vi "Decode IA_State.vi"(8 "error in (no error)":errorcluster, 11 "array":u8[](array[numeric])) -> (0 "error out":errorcluster, 3 "output cluster":T2)   [LabVIEW 2017]
uses:
  Util/Events/Events.ctl
panel:
  in  "?":T2={"Our_Robots"=[], "Events"={"Touch"=FALSE, "Ball out"=FALSE, "id touch"=0.0, "Ball out of \nVision"=FALSE, "Ball inside \nGoalie area"=FALSE, "Robot not responding"=FALSE, "Robots responding status"=[1.0, 1.0, 1.0, 1.0, 1.0, 1.0], "Enemy Ball \nPossession"=FALSE, "Pass State"=FALSE, "id end of pass"=0.0, "Kick"=FALSE, "Id ini Possession"=0.0, "Ball Possesion"=FALSE, "Id Possesion"=0.0}}
  out "array w/ subset deleted":u8[](array[numeric])
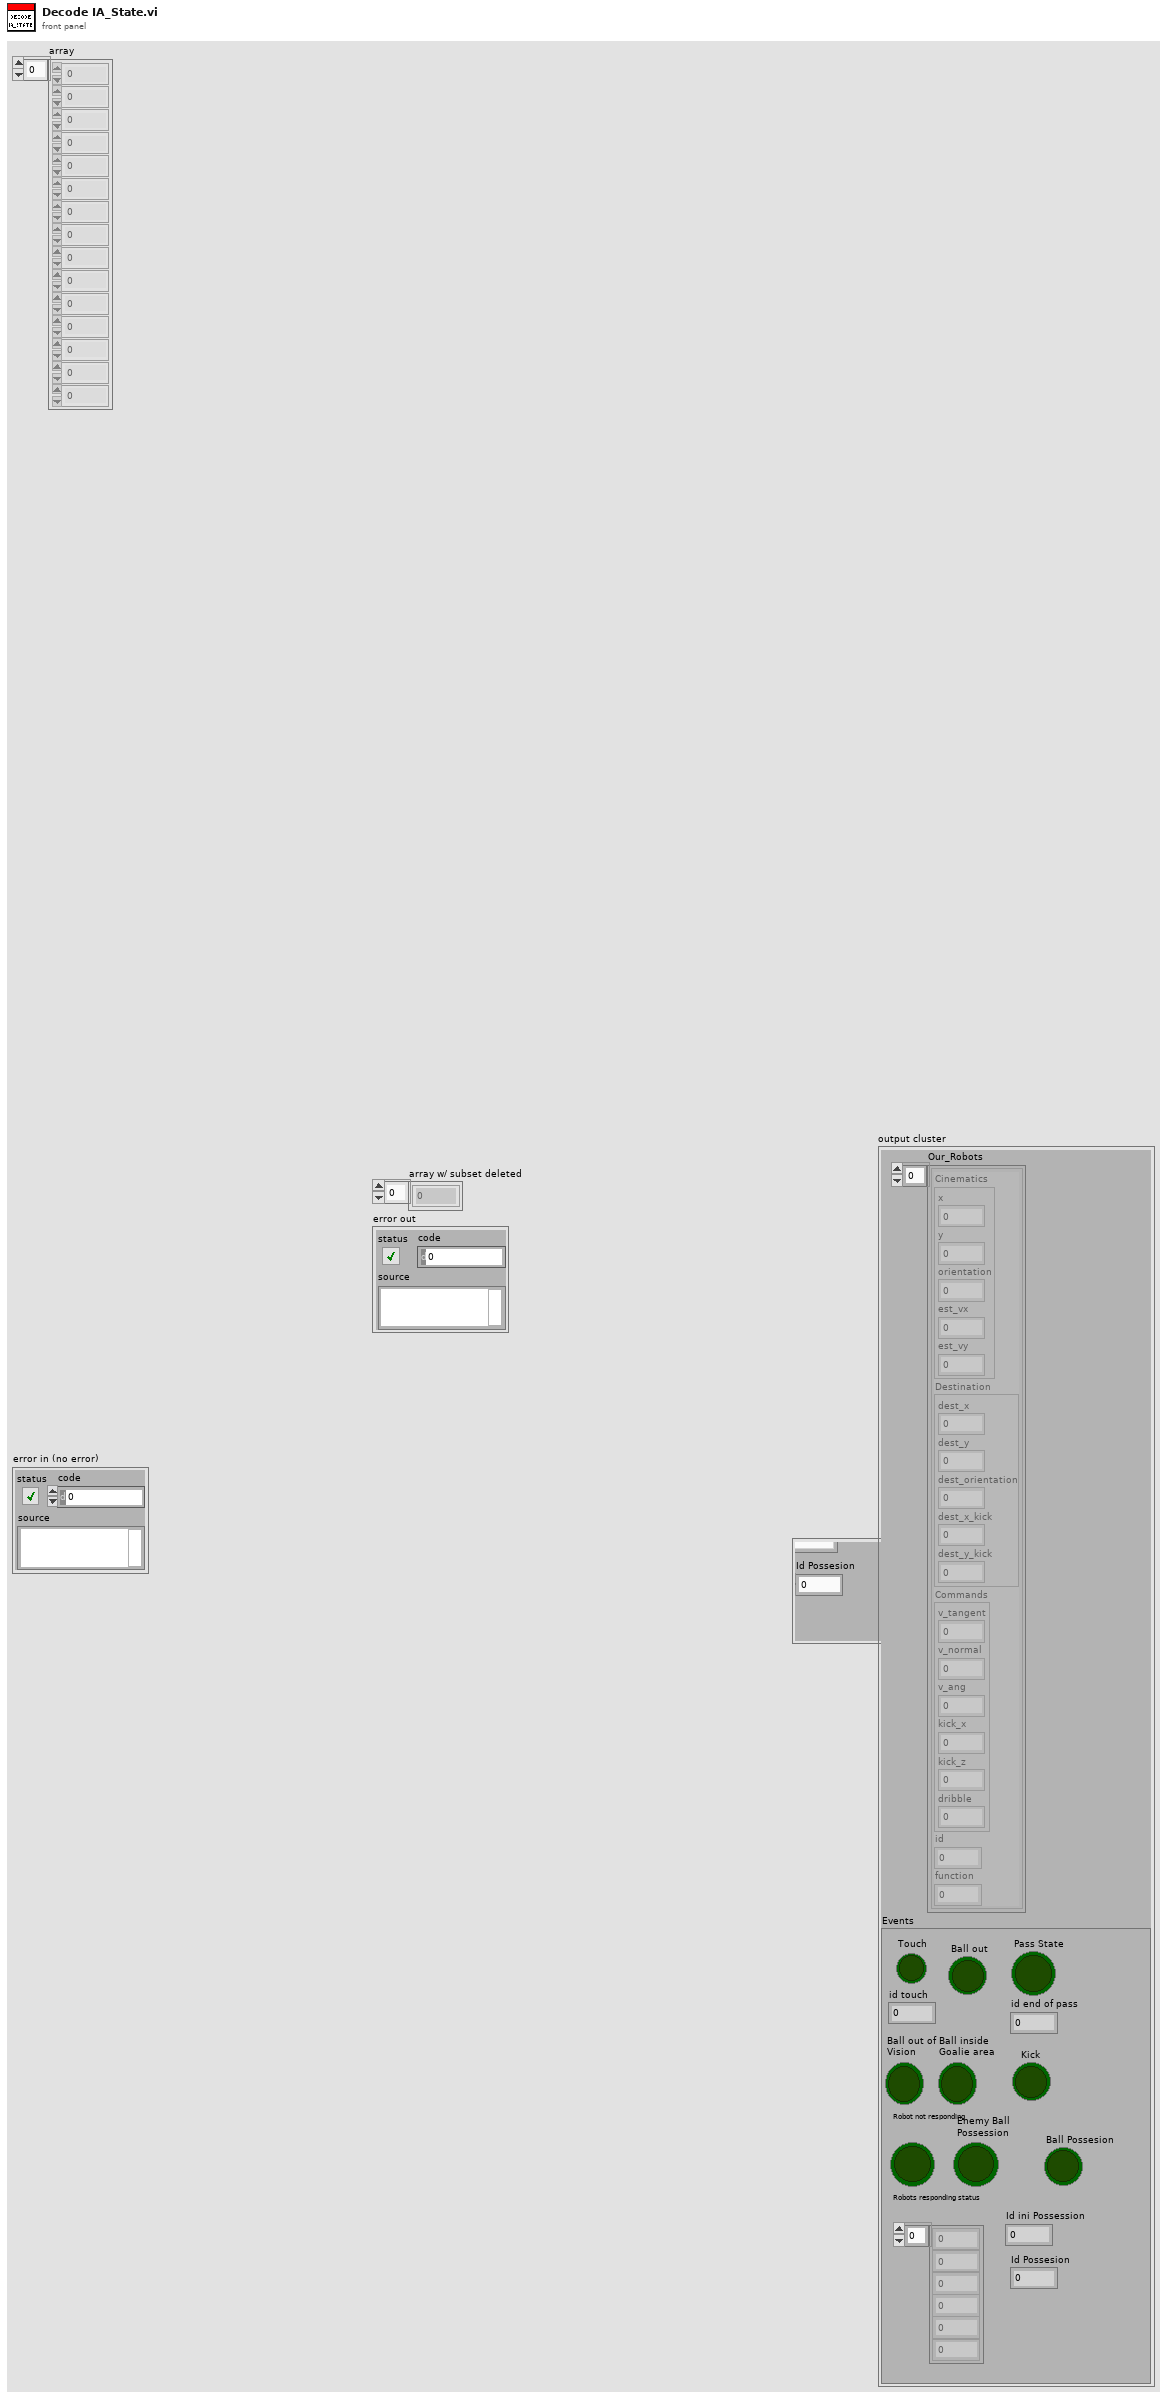
[diagram p1: front panel]
types:
  T1 = typedef "Events.ctl" = cluster{"Touch":bool, "Ball out":bool, "id touch":dbl, "Ball out of \nVision":bool, "Ball inside \nGoalie area":bool, "Robot not responding":bool, "Robots responding status":dbl[], "Enemy Ball \nPossession":bool, "Pass State":bool, "id end of pass":dbl, "Kick":bool, "Id ini Possession":dbl, "Ball Possesion":bool, "Id Possesion":dbl}
  T2 = cluster{"Our_Robots":cluster{"Cinematics":cluster{"x":dbl, "y":dbl, "orientation":dbl, "est_vx":dbl, "est_vy":dbl}, "Destination":cluster{"dest_x":dbl, "dest_y":dbl, "dest_orientation":dbl, "dest_x_kick":dbl, "dest_y_kick":dbl}, "Commands":cluster{"v_tangent":dbl, "v_normal":dbl, "v_ang":dbl, "kick_x":dbl, "kick_z":dbl, "dribble":u32}, "id":u32, "function":u32}[], "Events":T1}
  T3 = cluster{"Cinematics":cluster{"x":dbl, "y":dbl, "orientation":dbl, "est_vx":dbl, "est_vy":dbl}, "Destination":cluster{"dest_x":dbl, "dest_y":dbl, "dest_orientation":dbl, "dest_x_kick":dbl, "dest_y_kick":dbl}, "Commands":cluster{"v_tangent":dbl, "v_normal":dbl, "v_ang":dbl, "kick_x":dbl, "kick_z":dbl, "dribble":u32}, "id":u32, "function":u32}[]
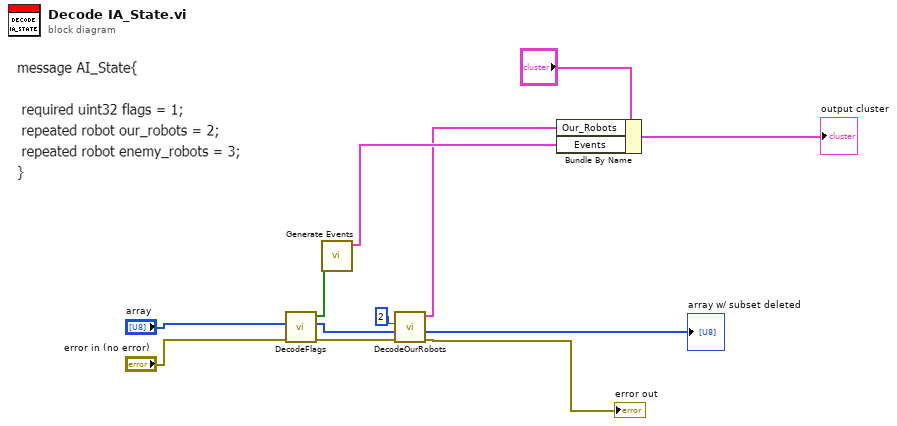
[diagram p0: block diagram]
diagram:
  n1 = call "DecodeFlags.vi"("error in"="error in (no error)", "Array"="array") -> ("error IO"=w9:errorcluster, "array w/ subset deleted"=w8:u8[], "Flags"=w12:bool[])  [unwired: 7 in]
  n2 = call "Generate Events.vi"("Flags"=w12) -> ("Events"=w3:T1)  [unwired: 10 in]
  n3 = call "DecodeOurRobots.vi"("error in"=w9, "array"=w8, "Key"=2) -> ("error out"=→"error out":errorcluster, "array w/ subset deleted out"=→"array w/ subset deleted":u8[], "Our_Robots"=w2:T3)  [unwired: 6 in]
  n4 = Bundle By Name(cluster="?", "Our_Robots"=w2, "Events"=w3) -> (→"output cluster":T2)
